vi "Create New Datafile.vi"(2 "Metadata":string="***** Metadata *****\nSample Description: Dummy\nCreator: Shivam\n", 3 "Filetype":u16(ring) items=[".xlsx", ".txt", ".csv"], 4 "File Base":path=path "C:/Users/qmgmit/Desktop/default_datafile.txt") -> (0 "Start time":timestamp=timestamp(3753397250.514444 s since 1904-01-01), 1 "File name":path=path "C:/Users/qmgmit/Desktop/Shivam/dev/dev/20221208_212050_newfile_vi.txt")   [LabVIEW 2020]
uses:
  <vilib>/Utility/file.llb/Write Delimited Spreadsheet (string).vi
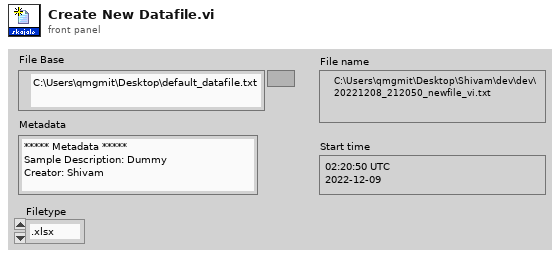
[diagram p1: front panel]
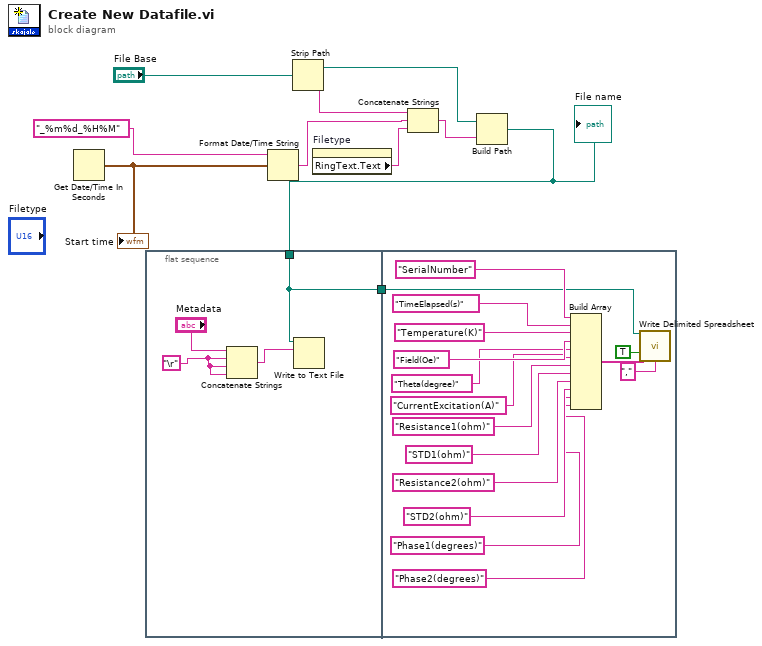
[diagram p0: block diagram]
diagram:
  n1 = Get Date/Time In Seconds() -> (seconds since 1Jan1904=w9:timestamp)
  "Start time" <- w9
  n2 = flat-sequence {
    tunnel: w5 -> [w12]
    tunnel: [w12] -> w4
    tunnel: w4 -> [w22]
    frame #0 {
      w11 = "\r"
      n3 = Concatenate Strings("Metadata", w11, w11, w11) -> (w13:string)
      n4 = Write to Text File(file (use dialog)=w12, text=w13) -> ()  [unwired: 2 in, 3 out]
    }
    frame #1 {
      n5 = Build Array("SerialNumber", "TimeElapsed(s)", "Temperature(K)", "Field(Oe)", "Theta(degree)", "CurrentExcitation(A)", "Resistance1(ohm)", "STD1(ohm)", "Resistance2(ohm)", "STD2(ohm)", "Phase1(degrees)", "Phase2(degrees)") -> (w30:string[])
      n6 = call-poly <vilib>:"Write Delimited Spreadsheet.vi"("file path (dialog if empty)"=w22, "1D data"=w30, "append to file? (new file:F)"=TRUE, "delimiter (\\t)"="," ("delimiter (\\t)")) -> ()  [unwired: 10 in, 2 out]
    }
  }
  n7 = Format Date/Time String(time format string (%c)="_%m%d_%H%M", seconds (now)=w9) -> (date/time string=w2:string)  [unwired: 1 in]
  n8 = Strip Path(path="File Base") -> (stripped path=w7:path, name=w3:string)
  n9 = property on="Filetype" class="Ring (strict)"() -> ("RingText.Text"=w1:string)  [unwired: 2 in, 2 out]
  n10 = Concatenate Strings(w3, w2, w1) -> (w6:string)
  n11 = Build Path(base path=w7, name or relative path=w6) -> (appended path=w5:path)
  "File name" <- w5
